vi "XIPIN_Reed-Solomon_Encoder_8_0.vi"   [LabVIEW 2017]
doc: "The Xilinx Reed-Solomon Encoder LogiCORE is a high speed, compact module that can be configured to implement many different Reed-Solomon coding standards. The core is fully synchronous, using a single clock, and supports continuous input data with no gap between code blocks. The core is parameterizable, allowing designers to control the symbol width and the code block length. The module supports shortened codes and any primitive field polynomial for a given symbol width. The core is delivered through the Xilinx CORE Generator System and integrates seamlessly with the Xilinx design flow.\n------------------------------------\n<b>Need License</b> : Yes\n<b>Interface</b> : AXI4-Stream"
uses:
  <vilib>/rvi/XilinxIP/XIPIN_XNode/niFpgaXIPIN.xnode
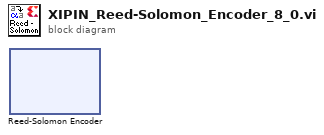
[diagram p0: block diagram]
diagram:
  n1 = xnode ("Reed-Solomon Encoder")() -> ()
